vi "Record Call.vi"(8 "error in (no error)":errorcluster, 10 "VI Name":string, 11 "One Of in":refnum<class "One Of.lvclass">) -> (0 "error out":errorcluster, 3 "One Of out":refnum<class "One Of.lvclass">)   [LabVIEW 2020, in "One Of.lvclass"]
uses:
  One Of.lvclass
  One Of.lvclass/One Of.ctl
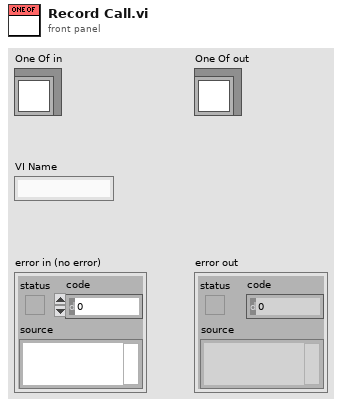
[diagram p1: front panel]
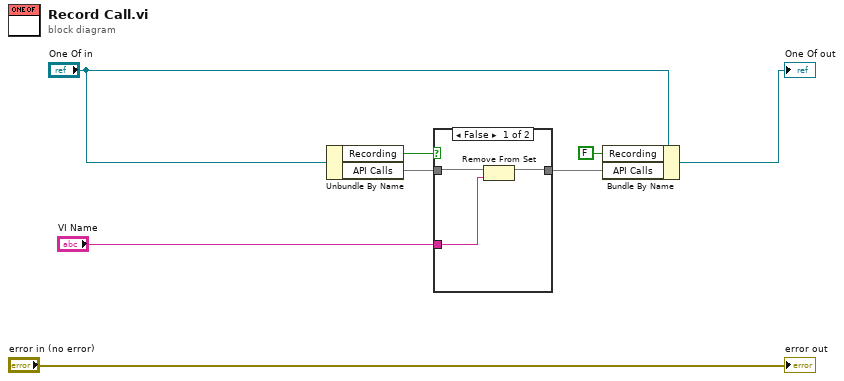
[diagram p0: block diagram]
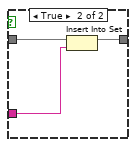
[diagram p2: hidden frame]
diagram:
  n1 = Unbundle By Name("One Of in") -> ("Recording"=w4:bool, "API Calls"=w7:set{string})
  n2 = case shown="False" w4 {
    tunnel: w7 -> [w11 w14]
    tunnel: "VI Name" -> [w10 w13]
    tunnel: [w9 w12] -> w6
    frame False {
      n3 = Remove From Set(10:w10, 11:w11) -> (3:w9:set{string})  [unwired: 1 out]
    }
    frame True {
      n4 = Insert Into Set(10:w13, 11:w14) -> (3:w12:set{string})  [unwired: 1 out]
    }
  }
  n5 = Bundle By Name(cluster="One Of in", "Recording"=FALSE, "API Calls"=w6) -> (→"One Of out":refnum<class "One Of.lvclass">)
  "error out" <- "error in (no error)"
